vi "Log_beam_power.vi"(3 "Message":string, 5 "Beam Data":dbl[][](array[numeric]) format="%.2f") -> ()   [LabVIEW 2010]
uses:
  Controls/Beam_Type.ctl
panel:
  out "Server copy Location":path
  out "Log File":path
  out "Beam Type":T1 items=["Green Unshifted", "Green Shifted", "Blue Unshifted", "Blue Shifted"]
  # "X                Y                 Z        Datum Power"
  # "Green Unshifted\nGreen Shifted\nBlue Unshifted\nBlue Shifted"
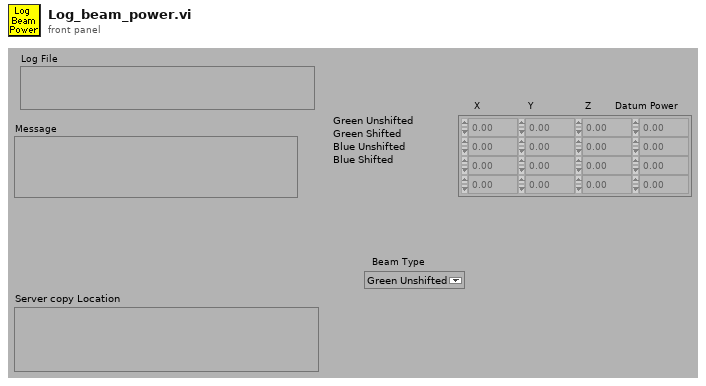
[diagram p1: front panel]
types:
  T1 = typedef "Beam_Type.ctl" = u16
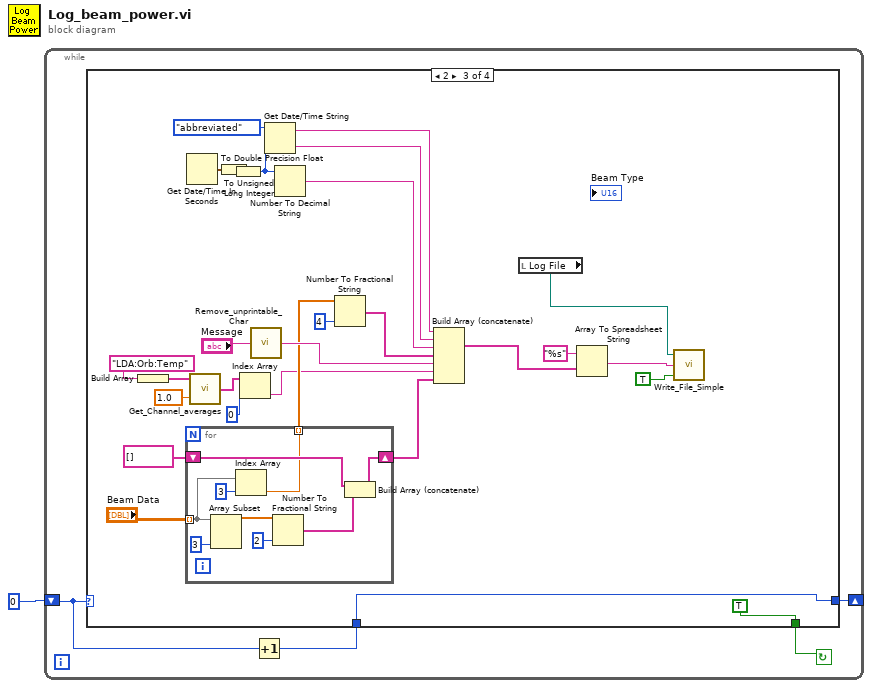
[diagram p0: block diagram]
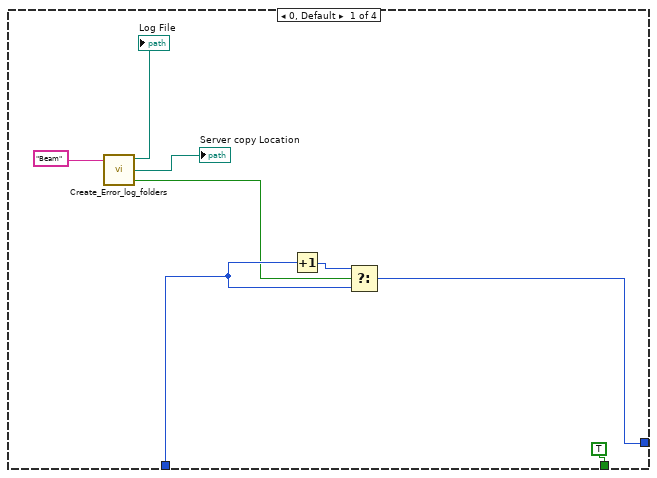
[diagram p2: hidden frame]
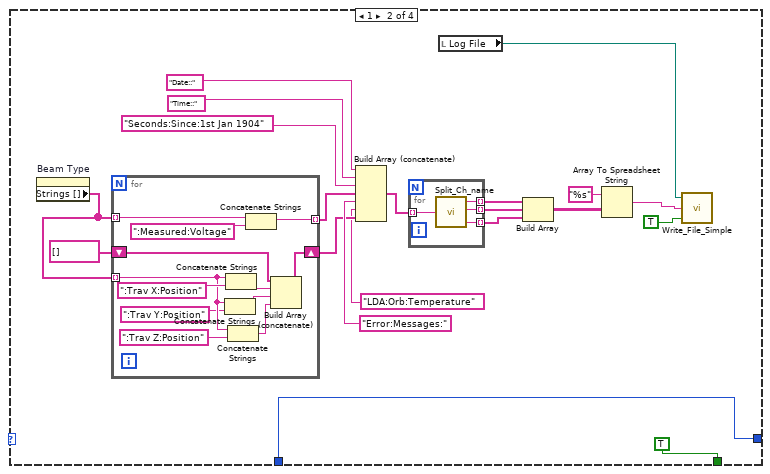
[diagram p3: hidden frame]
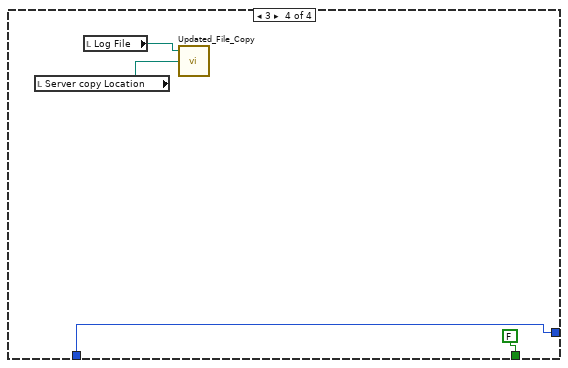
[diagram p4: hidden frame]
diagram:
  n1 = while {
    shift-left: 0 -> [w5]
    shift-right: [w2] -> _
    stop <- w4 continue-if-true
    n2 = Increment(x=w5) -> (x+1=w3:i32)
    n3 = case shown="2" w5 {
      tunnel: [TRUE TRUE TRUE FALSE] -> w4
      tunnel: w3 -> [w10 w21 w74 w87]
      tunnel: [w9 w21 w74 w87] -> w2
      frame 0, Default {
        n4 = call "Create_Error_log_folders.vi"("Log Filename"="Beam" ("Input Element")) -> ("exists?"=w7:bool, "Server copy Location"=→"Server copy Location":path, "Local Log File"=→"Log File":path)  [unwired: 2 in]
        n5 = Increment(x=w10) -> (x+1=w12:i32)
        n6 = Select(t=w12, s=w7, f=w10) -> (s? t:f=w9:i32)
      }
      frame 1 {
        n7 = property on="Beam Type" class="Ring (strict)"() -> ("Strings []"=w19:string[])  [unwired: 2 in, 2 out]
        n8 = for {
          tunnel: w19 -> [w45] mode=indexing
          tunnel: [w43] -> w24 mode=indexing
          shift-right: [w34] -> w18
          shift-left: string[] [] -> [w38]
          tunnel: w19 -> [w41] mode=indexing
          n9 = Concatenate Strings(w41, ":Trav Y:Position") -> (w36:string)
          n10 = Concatenate Strings(w41, ":Trav X:Position") -> (w37:string)
          n11 = Concatenate Strings(w41, ":Trav Z:Position") -> (w35:string)
          n12 = Concatenate Strings(w45, ":Measured:Voltage") -> (w43:string)
          n13 = Build Array (concatenate)(w38, w37, w36, w35) -> (w34:string[])
        }
        n14 = Build Array (concatenate)("Date::", "Time::", "Seconds:Since:1st Jan 1904", w24, "Error:Messages:", "LDA:Orb:Temperature", w18) -> (w27:string[])
        n15 = for {
          tunnel: w27 -> [w49] mode=indexing
          tunnel: [w48] -> w28 mode=indexing
          tunnel: [w47] -> w29 mode=indexing
          tunnel: [w46] -> w30 mode=indexing
          n16 = call "Split_Ch_name.vi"("Ch name"=w49) -> ("Top level"=w48:string, "Middle"=w47:string, "Low level"=w46:string)
        }
        n17 = local read "Log File"() -> (w14:path)
        n18 = Build Array(w28, w29, w30) -> (w25:string[][])
        n19 = Array To Spreadsheet String(array=w25, 3:"%s" ("format string")) -> (spreadsheet string=w15:string)  [unwired: 1 out]
        n20 = call "Write_File_Simple.vi"("append to file? (new file:F)"=TRUE, "character string"=w15, "file path"=w14) -> ()  [unwired: 2 out]
      }
      frame 2 {
        n21 = Build Array("LDA:Orb:Temp") -> (w58:string[])
        n22 = for {
          shift-right: [w85] -> w60
          shift-left: string[] [] -> [w86]
          tunnel: "Beam Data" -> [w79] mode=indexing
          tunnel: [w78] -> w61 mode=indexing
          n23 = Array Subset(array=w79, length=3 ("Array Length")) -> (w82:dbl[])  [unwired: 1 in]
          n24 = Index Array(array=w79, index=3 ("Index")) -> (element=w78:dbl)
          n25 = Number To Fractional String(number=w82, precision (6)=i16 2) -> (F-format string=w83:string[])  [unwired: 2 out]
          n26 = Build Array (concatenate)(w86, w83) -> (w85:string[])
        }
        n27 = Get Date/Time In Seconds() -> (seconds since 1Jan1904=w53:timestamp)
        n28 = call "Get_Channel_averages.vi"("Desired Ch Names"=w58, "Averaging time (mins)"=1.0) -> ("Values"=w56:string[])  [unwired: 1 in, 2 out]
        n29 = To Double Precision Float(number=w53) -> (double precision float=w72:dbl)
        n30 = To Unsigned Long Integer(number=w72) -> (unsigned 32bit integer=w71:u32)
        n31 = Index Array(array=w56, index=0 ("Index")) -> (element=w54:string)
        n32 = call "Remove_unprintable_Char.vi"("Input String"="Message") -> ("Output String"=w64:string)
        n33 = Get Date/Time String(date format (0)=enum16{"short", "long", "abbreviated"}."abbreviated", seconds (now)=w71) -> (date string=w70:string, time string=w69:string)  [unwired: 1 out]
        n34 = Number To Decimal String(number=w71) -> (decimal integer string=w68:string)  [unwired: 1 out]
        n35 = Number To Fractional String(number=w61, precision (6)=i16 4) -> (F-format string=w65:string[])  [unwired: 2 out]
        n36 = Build Array (concatenate)(w70, w69, w68, w65, w64, w54, w60) -> (w67:string[])
        n37 = local read "Log File"() -> (w50:path)
        n38 = Array To Spreadsheet String(array=w67, 3:"%s" ("format string")) -> (spreadsheet string=w51:string)  [unwired: 1 out]
        n39 = call "Write_File_Simple.vi"("append to file? (new file:F)"=TRUE, "character string"=w51, "file path"=w50) -> ()  [unwired: 2 out]
      }
      frame 3 {
        n40 = local read "Server copy Location"() -> (w89:path)
        n41 = local read "Log File"() -> (w90:path)
        n42 = call "Updated_File_Copy.vi"("Target Path"=w89, "Source Path"=w90) -> ()  [unwired: 2 out]
      }
    }
  }
